vi "StringifiedData.vi"(8 "error in (no error)":errorcluster, 11 "DoubleMsg in":refnum<class "DoubleMsg.lvclass">) -> (0 "error out":errorcluster, 2 "Stringified Data":string, 3 "DoubleMsg out":refnum<class "DoubleMsg.lvclass">)   [LabVIEW 2013, in "LapDog.Messaging.v3.NativeTypes.lvlib" / "DoubleMsg.lvclass"]
doc: "This VI is used for the message probe. Child classes may override it and provide the message data in string format or a short string describing the data the message contains. This string will be displayed in the probe window."
uses:
  DoubleMsg.lvclass
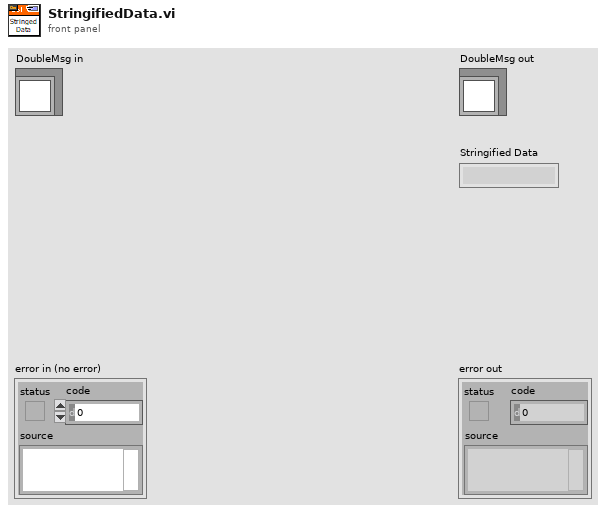
[diagram p1: front panel]
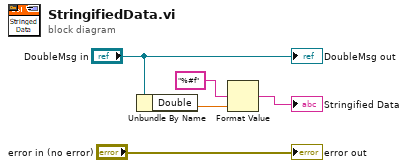
[diagram p0: block diagram]
diagram:
  n1 = Unbundle By Name("DoubleMsg in") -> ("Double"=w3:dbl)
  n2 = Format Value(format string="%#f", value (0)=w3) -> (output string=→"Stringified Data":string)  [unwired: 1 in]
  "error out" <- "error in (no error)"
  "DoubleMsg out" <- "DoubleMsg in"
